vi "No Grouped Tags.vi"(7 "caller name":string, 8 "error in (no error)":errorcluster, 11 "Empty List?":bool) -> (0 "error out":errorcluster)   [LabVIEW 2020, in "Current Value Table(Rebuild).lvlib"]
doc: "Throws an error if the input is an empty array."
uses:
  Current Value Table(Rebuild).lvlib
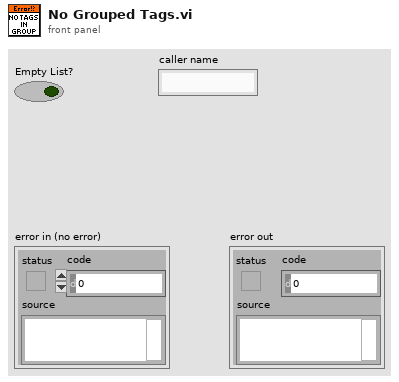
[diagram p1: front panel]
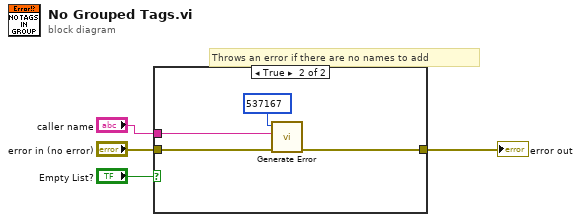
[diagram p0: block diagram]
diagram:
  # "Throws an error if there are no names to add"
  n1 = case shown="True" "Empty List?" {
    tunnel: "error in (no error)" -> [w5 w8]
    tunnel: [w5 w7] -> w4
    tunnel: "caller name" -> [_ w6]
    frame False {
    }
    frame True {
      n2 = call "Generate Error.vi"("error in"=w8, "caller name"=w6, "code"=537167) -> ("error out"=w7:errorcluster)  [unwired: 8 in]
    }
  }
  "error out" <- w4
